vi "Auto.vi"() -> ()   [LabVIEW 2020]
uses:
  <vilib>/Utility/miscctls.llb/LVRowAndColumnTypeDef.ctl
  Global_Variable/Global.vi
  Global_Variable/A131258.vi
  Database/Global1.vi
  <vilib>/addons/database/Connection.llb/DB Tools Open Connec (String).vi
  <vilib>/addons/database/Connection.llb/Conn Execute.vi
  <vilib>/addons/database/Recordset.llb/Rec Fetch Recordset Data (R).vi
  <vilib>/addons/database/NI_Database_API.lvlib
panel:
  out "标尺_Event":refnum<user-event>
  out "判定完成":bool=TRUE
  out "采集初始化":bool=TRUE
  out "左code":string
  out "初始化":bool[](array[boolean])
  out "空载":cluster{dbl[], dbl[]}[](graph)
  in  "判定结果":bool[][](array[boolean])=[[TRUE]]
  in  "STEP":string
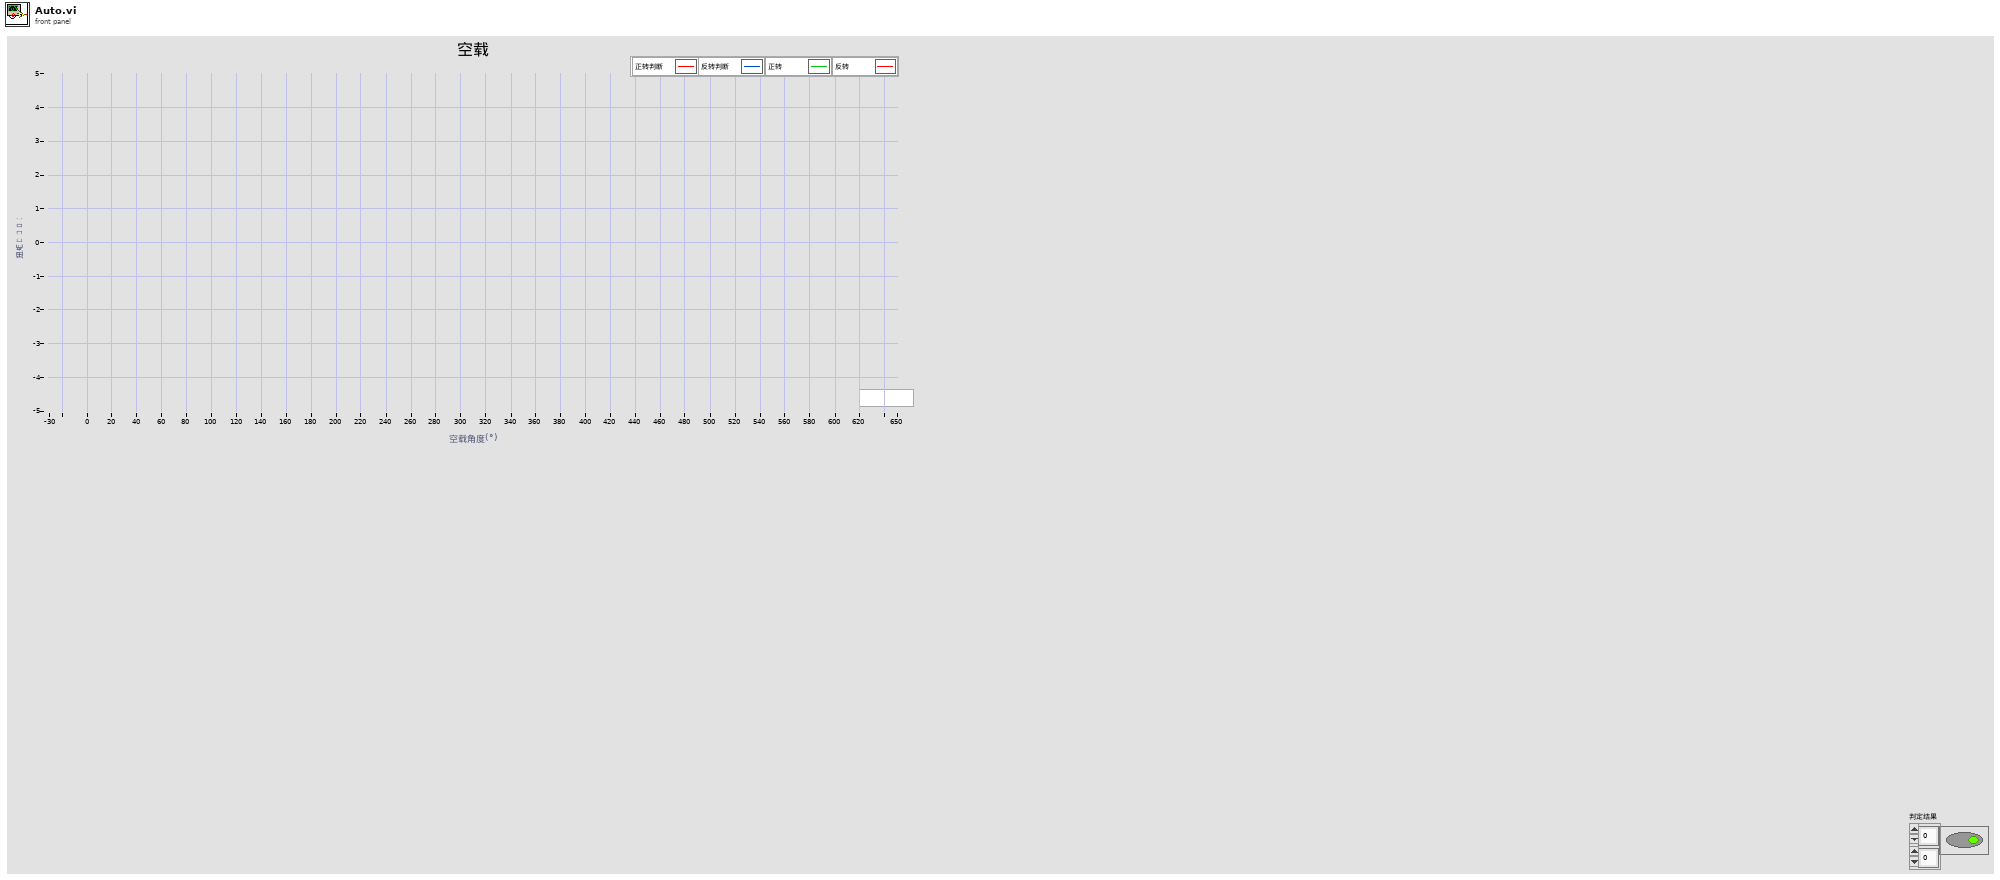
[diagram p1: front panel]
types:
  T1 = enum32{"Invalid", "Standard", "Closed", "Hidden", "Minimized", "Maximized"}
  T2 = typedef "LVRowAndColumnTypeDef.ctl" = cluster{"Row":i32, "Column":i32}
  T3 = typedef "lveventtype.ctl" = enum32{"Null", "Timeout", "Annotation Menu Selection", "Annotation Menu Selection?", "App Instance Close", "App Instance Close?", "Autoscale Range Change", "Bookmark Info Change", "Cell Edit", "Cell Edit?", "Cursor Grab", "Cursor Grab?", "Cursor Menu Selection", "Cursor Menu Selection?", "Cursor Move", "Cursor Release", "Data Change", "Direction Change", "Display State Change", "Drag Ended", "Drag Enter", "Drag Leave", "Drag Over", "Drag Source Update", "Drag Starting", "Drag Starting?", "Drop", "Exec State Change", "Key Down", "Key Down?", "Key Repeat", "Key Repeat?", "Key Up", "Listbox Double Click", "Menu Activation?", "Menu Selection (App)", "Menu Selection? (App)", "Menu Selection (User)", "Mouse Down", "Mouse Down?", "Mouse Enter", "Mouse Leave", "Mouse Move", "Mouse Up", "Mouse Wheel", "NI Security User Change (App)", "Pane Size", "Panel Close", "Panel Close?", "Panel Resize", "Plot Attribute Change", "Scale Range Change", "Shortcut Menu Activation?", "Shortcut Menu Selection (App)", "Shortcut Menu Selection? (App)", "Shortcut Menu Selection (User)", "Tree Double Click", "Tree Drag", "Tree Drag?", "Tree Drop", "Tree Drop?", "Tree Item Close", "Tree Item Close?", "Tree Item Open", "Tree Item Open?", "User Event", "Value Change"}
  T4 = typedef "LVPoint32TypeDef.ctl" = cluster{"Horizontal":i32, "Vertical":i32}
  T5 = cluster{"扭矩判定":cluster{"单位":string, "下限":dbl, "上限":dbl}, "正转扭矩最大值":cluster{"单位":string, "下限":dbl, "上限":dbl}, "正转扭矩最小值":cluster{"单位":string, "下限":dbl, "上限":dbl}, "正转扭矩波动值":cluster{"单位":string, "下限":dbl, "上限":dbl}, "正转平均扭矩值":cluster{"单位":string, "下限":dbl, "上限":dbl}, "反转扭矩最大值":cluster{"单位":string, "下限":dbl, "上限":dbl}, "反转扭矩最小值":cluster{"单位":string, "下限":dbl, "上限":dbl}, "反转扭矩波动值":cluster{"单位":string, "下限":dbl, "上限":dbl}, "反转扭矩平均值":cluster{"单位":string, "下限":dbl, "上限":dbl}, "正/逆转平均扭矩差":cluster{"单位":string, "下限":dbl, "上限":dbl}}
  T6 = cluster{"正向判定X值":cluster{"单位":string, "下限":dbl, "上限":dbl}, "正向判定Y值":cluster{"单位":string, "下限":dbl, "上限":dbl}, "逆向判定X值":cluster{"单位":string, "下限":dbl, "上限":dbl}, "逆向判定Y值":cluster{"单位":string, "下限":dbl, "上限":dbl}}
  T7 = cluster{"左平均扭矩":cluster{"正转":dbl, "反转":dbl}, "左矩波动":cluster{"正转":dbl, "反转":dbl}, "左空载":cluster{"正转":dbl, "反转":dbl}, "右平均扭矩":cluster{"正转":dbl, "反转":dbl}, "右扭矩波动":cluster{"正转":dbl, "反转":dbl}, "右空载":cluster{"正转":dbl, "反转":dbl}, "扭矩对称":cluster{"左":dbl, "右":dbl}, "左零点漂移":cluster{"正":dbl, "反":dbl}, "右零点漂移":cluster{"正":dbl, "反":dbl}}
  T8 = typedef "NI_Database_API.lvlib/Conn ObjectReference.ctl" = refnum<k1>
  T9 = typedef "NI_Database_API.lvlib/Rec ObjectReference.ctl" = refnum<k1>
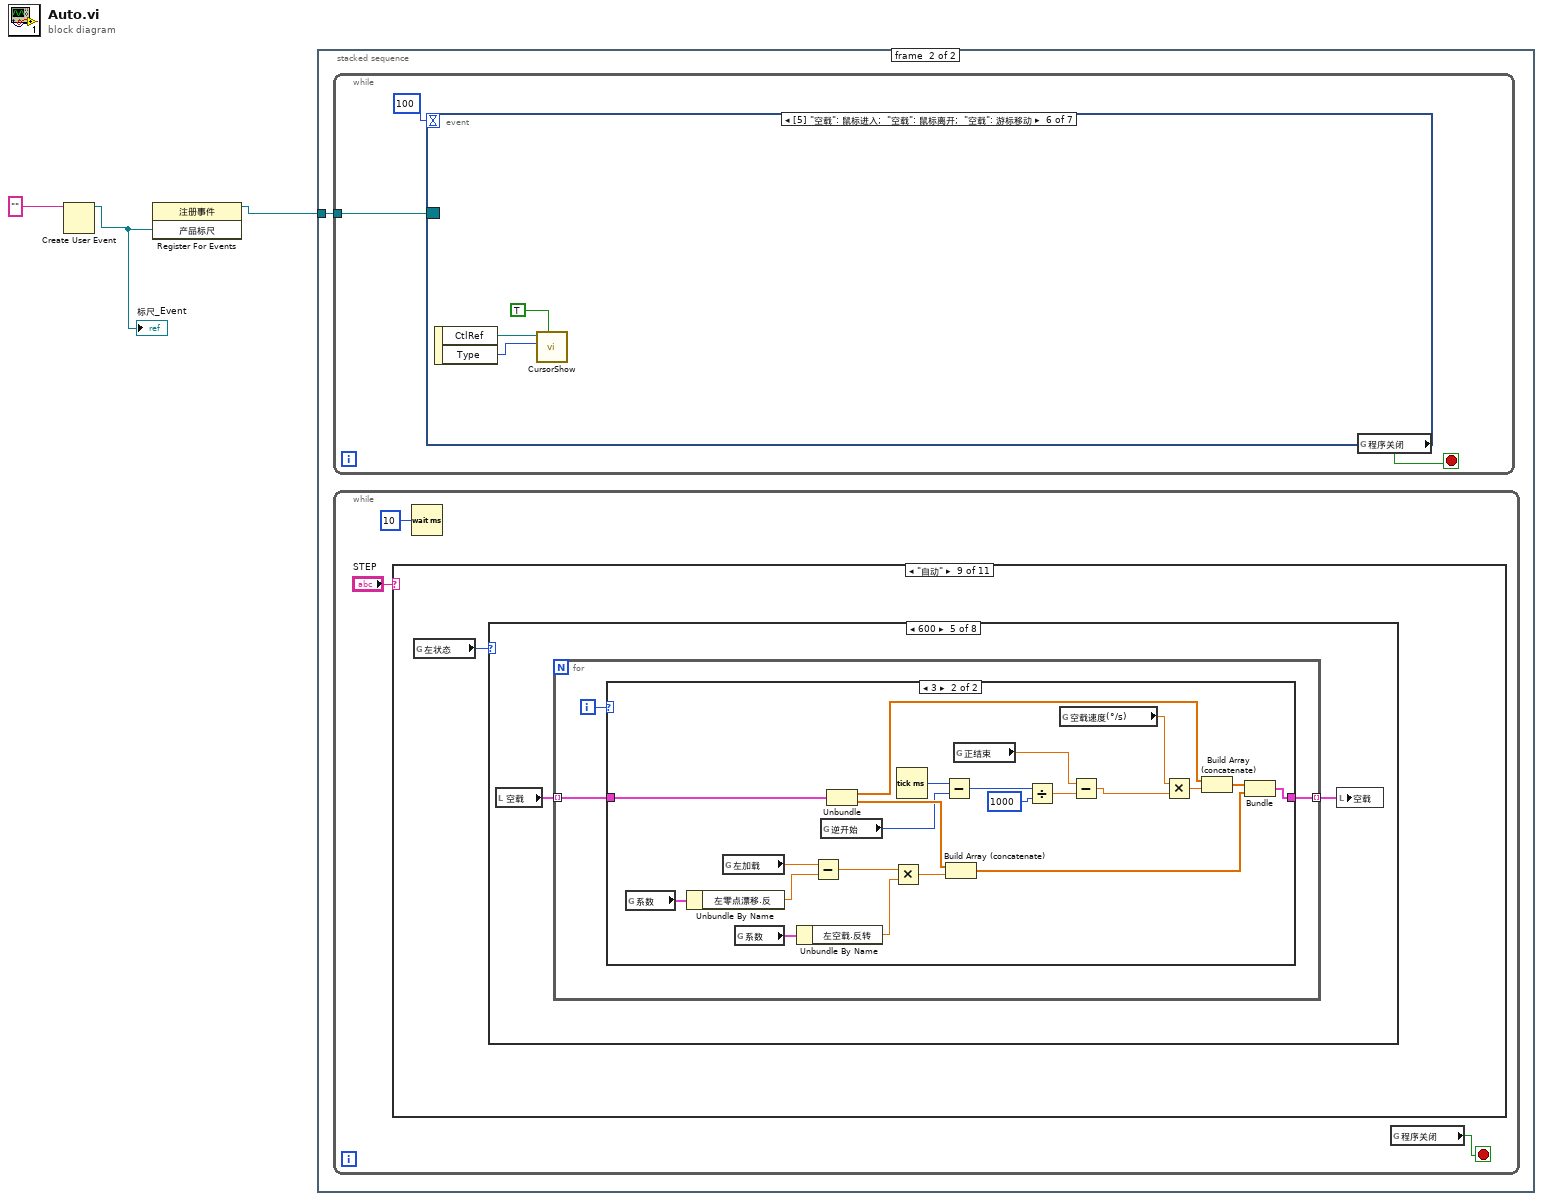
[diagram p0: block diagram]
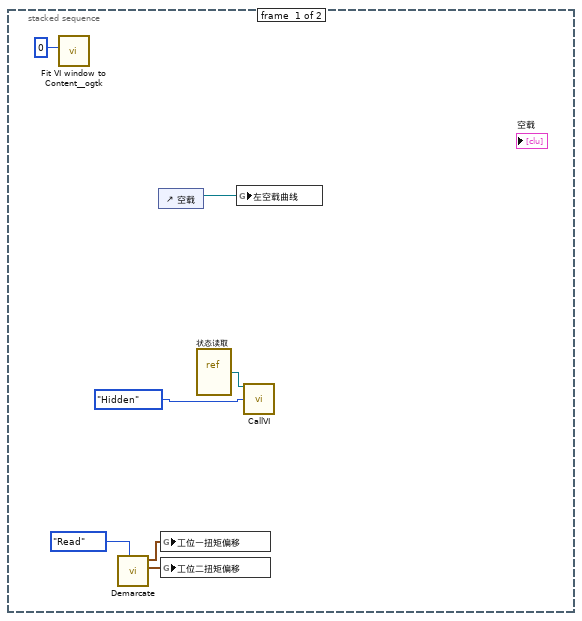
[diagram p2: hidden frame]
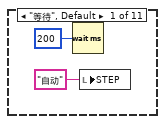
[diagram p3: hidden frame]
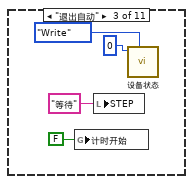
[diagram p5: hidden frame]
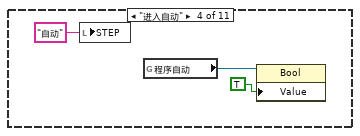
[diagram p6: hidden frame]
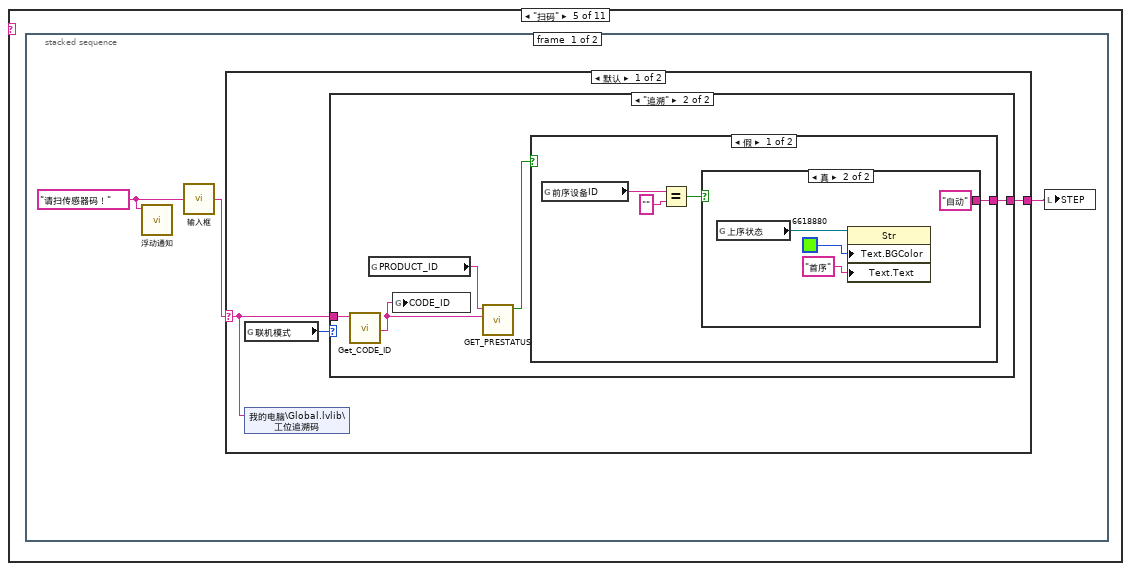
[diagram p7: hidden frame]
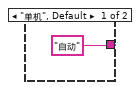
[diagram p8: hidden frame]
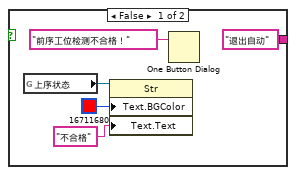
[diagram p9: hidden frame]
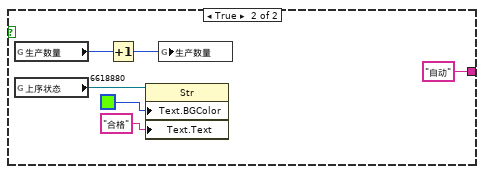
[diagram p10: hidden frame]
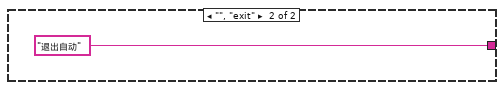
[diagram p11: hidden frame]
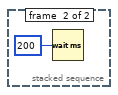
[diagram p12: hidden frame]
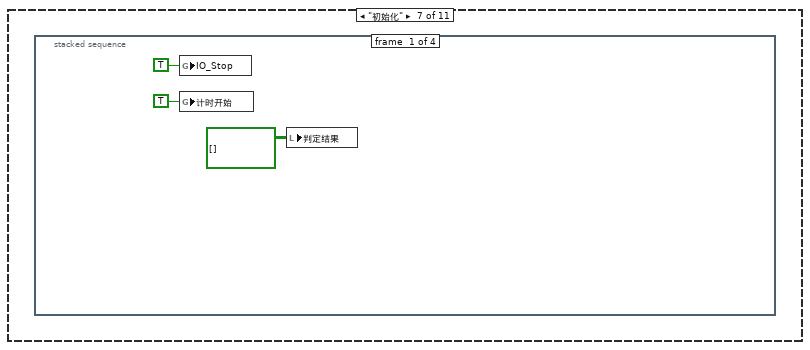
[diagram p14: hidden frame]
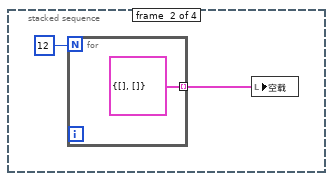
[diagram p15: hidden frame]
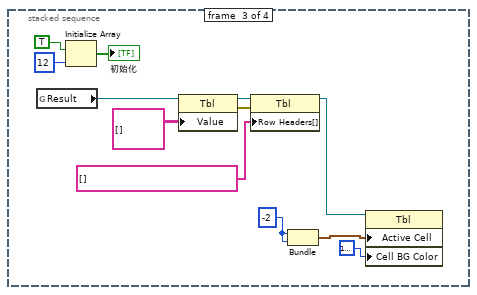
[diagram p16: hidden frame]
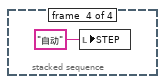
[diagram p17: hidden frame]
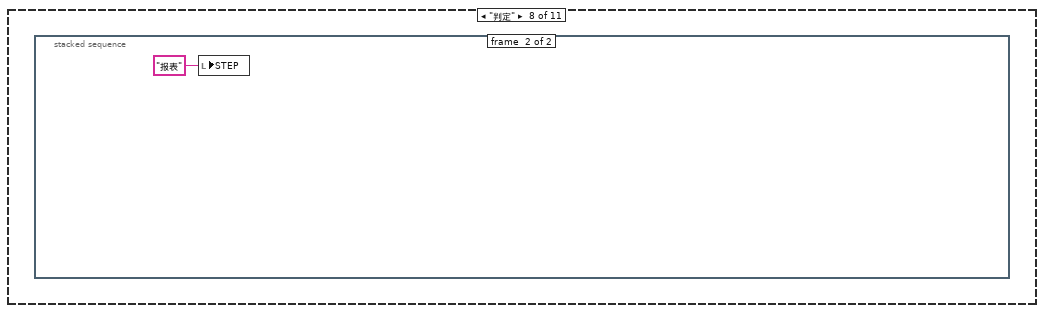
[diagram p18: hidden frame]
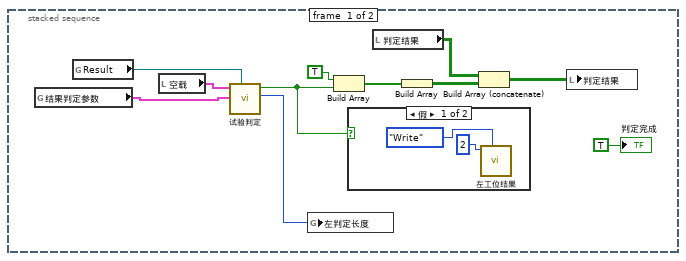
[diagram p19: hidden frame]
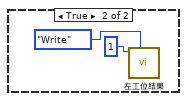
[diagram p20: hidden frame]
diagram:
  n1 = Create User Event(user event datatype="" ("产品标尺")) -> (user event=w2:refnum<user-event>)  [unwired: 1 in, 1 out]
  "标尺_Event" <- w2
  n2 = register-events(w2) -> (reference out=w1:refnum<event-registration>)  [unwired: 2 in, 1 out]
  n3 = stacked-sequence {
    tunnel: w1 -> [_ w11]
    frame #0 {
      n4 = call <userlib>:"Fit VI window to Content__ogtk.vi"("border spacing (2 px)"=0) -> ()  [unwired: 5 in, 2 out]
      n5 = call "Demarcate.vi"("Mode"=enum16{"Read", "Write"}."Read") -> ("工位二扭矩偏移O"=w5:cluster{"正向":dbl, "逆向":dbl}, "工位一扭矩偏移O"=w6:cluster{"正向":dbl, "逆向":dbl})  [unwired: 8 in, 1 out]
      n6 = control-ref of="空载"() -> (w4:refnum<vi>)
      n7 = global write "Global.vi" "工位一扭矩偏移"(w6) -> ()
      n8 = global write "Global.vi" "工位二扭矩偏移"(w5) -> ()
      n9 = vi-ref "状态读取.vi"() -> (w9:refnum<vi>)
      n10 = global write "A131258.vi" "左空载曲线"(w4) -> ()
      n11 = call "CallVI.vi"("VI引用"=w9, "状态"=T1."Hidden") -> ()  [unwired: 11 in, 3 out]
    }
    frame #1 {
      n12 = while {
        tunnel: w11 -> [w327]
        stop <- w328 stop-if-true
        n13 = event shown="[5] \"空载\": 鼠标进入;  \"空载\": 鼠标离开;  \"空载\": 游标移动" {
          selector: w327 -> [_ _ _ _ _ _ _]
          dyn-events: _ -> [_ _ _ _ _ _ _]
          timeout: 100 -> [_ _ _ _ _ _ _]
          event Timeout {
            n14 = event-data() -> ()  [unwired: 1 in, 3 out]
            n15 = global read "Global.vi" "跳转"() -> (w330:i16)
            n16 = case shown="1001" w330 {
              frame 0, Default {
              }
              frame 1000 {
                w334 = "" ("文本.文本")
                n17 = shared-variable "我的电脑\\Global.lvlib\\总成追溯码"(w334) -> ()  [unwired: 1 in, 1 out]
                n18 = shared-variable "我的电脑\\Global.lvlib\\工位追溯码"(w334) -> ()  [unwired: 1 in, 1 out]
                n19 = shared-variable "我的电脑\\Global.lvlib\\传感器码-左"(w334) -> ()  [unwired: 1 in, 1 out]
                n20 = shared-variable "我的电脑\\Global.lvlib\\传感器码-右"(w334) -> ()  [unwired: 1 in, 1 out]
                n21 = local write "STEP"("扫码" ("STEP")) -> ()
                n22 = call "跳转步骤.vi"("枚举"=enum16{"Read", "Write"}."Write", "Status_Write"=u16 1001 ("跳转步骤")) -> ()  [unwired: 9 in, 1 out]
              }
              frame 1001 {
                n23 = global read "Global.vi" "左在位"() -> (w335:i16)
                n24 = case shown="1" w335 {
                  frame 0, Default {
                  }
                  frame 1 {
                    w338 = enum16{"Read", "Write"}."Write" ("枚举")
                    n25 = local write "STEP"("自动" ("STEP")) -> ()
                    n26 = call "左工位状态.vi"("枚举"=w338, "Status_Write"=u16 1001 ("左工位状态")) -> ()  [unwired: 9 in, 1 out]
                    n27 = call "左工位在位.vi"("枚举"=w338, "Status_Write"=u16 0 ("左工位工件在位")) -> ()  [unwired: 9 in, 1 out]
                  }
                }
              }
            }
          }
          event Menu Selection (User) {
            n28 = event-data() -> ("ItemTag"=w340:string)  [unwired: 1 in, 2 out]
            n29 = case shown="\"假\", 默认" w340 {
              frame "假", Default {
              }
              frame "真" {
              }
            }
          }
          event "空载": Scale Range Change {
            n30 = event-data() -> ("CtlRef"=w343:refnum<vi>)  [unwired: 1 in]
            n31 = shared-variable "我的电脑\\Global.lvlib\\产品型号"() -> (w341:string)  [unwired: 1 in, 1 out]
            n32 = call "XY_conf.vi"("方式"=enum16{"写入", "读取"}."写入", "产品型号"=w341, "XY图引用"=w343) -> ()  [unwired: 3 in, 1 out]
          }
          event User Event {
            n33 = event-data() -> ("产品标尺"=w346:string)  [unwired: 1 in, 4 out]
            n34 = control-ref of="空载"() -> (w344:refnum<vi>)
            n35 = call "XY_conf.vi"("方式"=enum16{"写入", "读取"}."读取", "产品型号"=w346, "XY图引用"=w344) -> ()  [unwired: 3 in, 1 out]
          }
          event Panel Close {
            n36 = event-data() -> ()  [unwired: 1 in, 4 out]
            n37 = global write "Global.vi" "程序关闭"(TRUE ("程序关闭")) -> ()
          }
          event "空载": Mouse Enter; "空载": Mouse Leave; "空载": Cursor Move {
            n38 = event-data() -> ("CtlRef"=w350:refnum<vi>, "Type"=w348:T3)  [unwired: 1 in]
            n39 = call "CursorShow.vi"("nameShow"=TRUE, "Type"=w348, "Graph"=w350) -> ()  [unwired: 7 in, 2 out]
          }
          event "空载": Mouse Down {
            n40 = event-data() -> ("CtlRef"=w355:refnum<vi>, "Coords"=w354:T4, "Type"=w352:T3)  [unwired: 1 in]
            n41 = invoke class="XYGraph (严格)" method="Map Coords To XY"(reference=w355, "Coords"=w354) -> (reference out=w353:refnum<vi>, "XY"=w351:cluster{"X":dbl, "Y":dbl})  [unwired: 5 in, 5 out]
            n42 = call "CursorShow.vi"("游标.游标位置"=w351, "Type"=w352, "Graph"=w353) -> ()  [unwired: 7 in, 2 out]
          }
        }
        n43 = global read "Global.vi" "程序关闭"() -> (w328:bool)
      }
      n44 = while {
        stop <- w14 stop-if-true
        n45 = case shown="\"自动\"" "STEP" {
          frame "等待", Default {
            n46 = Wait (ms)(milliseconds to wait=u32 200 ("等待时间（毫秒）")) -> ()  [unwired: 1 out]
            n47 = local write "STEP"("自动" ("STEP")) -> ()
          }
          frame "手动" {
          }
          frame "退出自动" {
            n48 = global write "Global.vi" "计时开始"(FALSE ("计时开始")) -> ()
            n49 = local write "STEP"("等待" ("STEP")) -> ()
            n50 = call "设备状态.vi"("枚举"=enum16{"Read", "Write"}."Write", "Status_Write"=i16 0) -> ()  [unwired: 9 in, 1 out]
          }
          frame "进入自动" {
            n51 = local write "STEP"("自动" ("STEP")) -> ()
            n52 = global read "Global.vi" "程序自动"() -> (w22:refnum<vi>)
            n53 = property class="Bool"(reference=w22, "Value"=TRUE) -> ()  [unwired: 1 in, 2 out]
          }
          frame "扫码" {
            n54 = stacked-sequence {
              frame #0 {
                w25 = "请扫传感器码！" ("提示信息")
                n55 = call "浮动通知.vi"("通知内容"=w25) -> ()  [unwired: 11 in]
                n56 = call "输入框.vi"("提示信息"=w25) -> ("条形码输出"=w26:string)
                n57 = case shown="默认" w26 {
                  selector: w26 -> [w27 _]
                  tunnel: [w29 "退出自动" ("State(s) in Front (\"\")")] -> w24
                  frame Default {
                    n58 = global read "Global1.vi" "联机模式"() -> (w28:enum16{"单机", "追溯"})
                    n59 = shared-variable "我的电脑\\Global.lvlib\\工位追溯码"(w27) -> ()  [unwired: 1 in, 1 out]
                    n60 = case shown="\"追溯\"" w28 {
                      tunnel: ["自动" ("State(s) in Front (\"\")") w35] -> w29
                      tunnel: w27 -> [_ w34]
                      frame "单机", Default {
                      }
                      frame "追溯" {
                        n61 = call "Get_CODE_ID.vi"("CODE_MAIN"=w34) -> ("CODE_ID"=w31:string)  [unwired: 10 in]
                        n62 = global read "追溯Global.vi" "PRODUCT_ID"() -> (w33:string)
                        n63 = global write "追溯Global.vi" "CODE_ID"(w31) -> ()
                        n64 = call "GET_PRESTATUS.vi"("CODE_ID"=w31, "PRODUCT_ID"=w33) -> ("OK?"=w32:bool)  [unwired: 8 in, 1 out]
                        n65 = case shown="假" w32 {
                          tunnel: [w39 "自动" ("State(s) in Front (\"\")")] -> w35
                          frame False {
                            n66 = global read "追溯Global.vi" "前序设备ID"() -> (w38:string)
                            n67 = Equal?(x=w38, y="") -> (x = y?=w37:bool)
                            n68 = case shown="真" w37 {
                              tunnel: ["退出自动" ("State(s) in Front (\"\")") "自动" ("State(s) in Front (\"\")")] -> w39
                              frame False {
                                n69 = global read "Global.vi" "上序状态"() -> (w42:refnum<vi>)
                                n70 = property class="Str"(reference=w42, "Text.BGColor"=u32 16711680 ("文本.文本颜色:背景色"), "Text.Text"="不合格" ("文本.文本")) -> ()  [unwired: 1 in, 2 out]
                                n71 = One Button Dialog(message="前序工位检测不合格！" ("消息")) -> ()  [unwired: 1 in, 1 out]
                              }
                              frame True {
                                n72 = global read "Global.vi" "上序状态"() -> (w47:refnum<vi>)
                                n73 = property class="Str"(reference=w47, "Text.BGColor"=u32 6618880 ("文本.文本颜色:背景色"), "Text.Text"="首序" ("文本.文本")) -> ()  [unwired: 1 in, 2 out]
                              }
                            }
                          }
                          frame True {
                            n74 = global read "Global.vi" "生产数量"() -> (w52:i32)
                            n75 = global read "Global.vi" "上序状态"() -> (w51:refnum<vi>)
                            n76 = Increment(x=w52) -> (x+1=w53:i32)
                            n77 = property class="Str"(reference=w51, "Text.BGColor"=u32 6618880 ("文本.文本颜色:背景色"), "Text.Text"="合格" ("文本.文本")) -> ()  [unwired: 1 in, 2 out]
                            n78 = global write "Global.vi" "生产数量"(w53) -> ()
                          }
                        }
                      }
                    }
                  }
                  frame "", "exit" {
                  }
                }
                n79 = local write "STEP"(w24) -> ()
              }
              frame #1 {
                n80 = Wait (ms)(milliseconds to wait=u32 200 ("等待时间（毫秒）")) -> ()  [unwired: 1 out]
              }
            }
          }
          frame "工位判断" {
          }
          frame "初始化" {
            n81 = stacked-sequence {
              frame #0 {
                n82 = global write "Global.vi" "IO_Stop"(TRUE ("IO_Stop")) -> ()
                n83 = global write "Global.vi" "计时开始"(TRUE ("计时开始")) -> ()
                n84 = local write "判定结果"(bool[][] [] ("判定结果")) -> ()
              }
              frame #1 {
                n85 = for {
                  N: 12 -> [_]
                  tunnel: [cluster{dbl[], dbl[]} {[], []}] -> w60 mode=indexing
                }
                n86 = local write "空载"(w60) -> ()
              }
              frame #2 {
                w63 = -2 ("维数大小")
                n87 = global read "Global.vi" "Result"() -> (w72:refnum<vi>)
                n88 = Initialize Array(TRUE, 12 ("维数大小")) -> (→"初始化":bool[])
                n89 = property class="Tbl"(reference=w72, "Value"=string[][] []) -> (reference out=w73:refnum<vi>, error out=w74:errorcluster)  [unwired: 1 in]
                n90 = property class="Tbl"(reference=w73, error in=w74, "Row Headers[]"=string[] [] ("列首字符串[]")) -> (reference out=w66:refnum<vi>)  [unwired: 1 out]
                n91 = Bundle("维数大小"=w63, "维数大小"=w63) -> (w64:cluster{"维数大小":i32, "维数大小":i32})  [unwired: 1 in]
                n92 = property class="Tbl"(reference=w66, "Active Cell"=w64, "Cell BG Color"=u32 16777216 ("活动单元格:单元格背景色")) -> ()  [unwired: 1 in, 2 out]
              }
              frame #3 {
                n93 = local write "STEP"("自动" ("STEP")) -> ()
              }
            }
          }
          frame "判定" {
            n94 = stacked-sequence {
              frame #0 {
                n95 = global read "A131258.vi" "结果判定参数"() -> (w78:T5)
                n96 = global read "Global.vi" "Result"() -> (w80:refnum<vi>)
                n97 = local read "空载"() -> (w79:cluster{dbl[], dbl[]}[])
                n98 = call "试验判定.vi"("Result"=w80, "判定参数"=w78, "XY曲线"=w79) -> ("判定项长度"=w77:i32, "OK？"=w81:bool)  [unwired: 7 in]
                n99 = global write "判定参数.vi" "左判定长度"(w77) -> ()
                n100 = Build Array(TRUE ("元素"), w81) -> (w84:bool[])
                n101 = case shown="假" w81 {
                  frame False {
                    n102 = call "左工位结果.vi"("枚举"=enum16{"Read", "Write"}."Write", "Status_Write"=u16 2 ("左工位生产结果")) -> ()  [unwired: 9 in, 1 out]
                  }
                  frame True {
                    n103 = call "左工位结果.vi"("枚举"=enum16{"Read", "Write"}."Write", "Status_Write"=u16 1 ("左工位生产结果")) -> ()  [unwired: 9 in, 1 out]
                  }
                }
                n104 = local read "判定结果"() -> (w85:bool[][])
                n105 = Build Array(w84) -> (w83:bool[][])
                n106 = Build Array (concatenate)(w85, w83) -> (w86:bool[][])
                n107 = local write "判定结果"(w86) -> ()
                "判定完成" <- TRUE
              }
              frame #1 {
                n108 = local write "STEP"("报表" ("STEP")) -> ()
              }
            }
          }
          frame "自动" {
            n109 = global read "Global.vi" "左状态"() -> (w92:i16)
            n110 = case shown="600" w92 {
              frame 0, Default {
              }
              frame 3 {
                n111 = stacked-sequence {
                  frame #0 {
                    n112 = local write "判定结果"(bool[][] [] ("判定结果")) -> ()
                    n113 = call "左工位结果.vi"("枚举"=enum16{"Read", "Write"}."Write", "Status_Write"=i16 0) -> ()  [unwired: 9 in, 1 out]
                  }
                  frame #1 {
                    n114 = global read "Global.vi" "空载速度(°/s) 2"() -> (w96:sgl)
                    n115 = Multiply(x=w96, y=sgl 6.0) -> (x*y=w97:sgl)
                    n116 = global write "Global.vi" "空载速度(°/s)"(w97) -> ()
                  }
                }
              }
              frame 200 {
                n117 = stacked-sequence {
                  frame #0 {
                    n118 = local write "判定完成"(FALSE ("判定完成")) -> ()
                    n119 = call "左工位结果.vi"("枚举"=enum16{"Read", "Write"}."Write", "Status_Write"=u16 0 ("左工位生产结果")) -> ()  [unwired: 9 in, 1 out]
                    "采集初始化" <- TRUE
                  }
                  frame #1 {
                    n120 = for {
                      N: 4 -> [_]
                      tunnel: [cluster{dbl[], dbl[]} {[], []}] -> w104 mode=indexing
                    }
                    n121 = local write "空载"(w104) -> ()
                  }
                  frame #2 {
                    n122 = global read "Global.vi" "Result"() -> (w110:refnum<vi>)
                    n123 = property class="Tbl"(reference=w110, "Row Headers[]"=string[] [] ("行首字符串[]"), "Value"=string[][] [] ("值"), "Active Cell"=T2 {"Row"=-2, "Column"=-2} ("活动单元格:活动单元格"), "Cell BG Color"=u32 16777216 ("活动单元格:单元格背景色")) -> ()  [unwired: 1 in, 2 out]
                  }
                  frame #3 {
                    n124 = local read "空载"() -> (w111:cluster{dbl[], dbl[]}[])
                    n125 = for {
                      tunnel: [w114] -> w112 mode=indexing
                      tunnel: w111 -> [w113] mode=indexing
                      i -> [w115]
                      n126 = case shown="1" w115 {
                        tunnel: [w116 w117 w125] -> w114
                        tunnel: w113 -> [w116 _ _]
                        frame Default {
                        }
                        frame 0 {
                          n127 = global read "A131258.vi" "判定框参数"() -> (w122:T6)
                          n128 = Unbundle By Name(w122) -> ("正向判定X值.下限"=w121:dbl, "正向判定X值.上限"=w120:dbl, "正向判定Y值.下限"=w119:dbl, "正向判定Y值.上限"=w118:dbl)
                          n129 = Build Array(w120, w120, w121, w121, w120) -> (w124:dbl[])
                          n130 = Build Array(w118, w119, w119, w118, w118) -> (w123:dbl[])
                          n131 = Bundle(w124, w123) -> (w117:cluster{dbl[], dbl[]})  [unwired: 1 in]
                        }
                        frame 1 {
                          n132 = global read "A131258.vi" "判定框参数"() -> (w130:T6)
                          n133 = Unbundle By Name(w130) -> ("逆向判定X值.下限"=w129:dbl, "逆向判定X值.上限"=w128:dbl, "逆向判定Y值.下限"=w127:dbl, "逆向判定Y值.上限"=w126:dbl)
                          n134 = Build Array(w128, w128, w129, w129, w128) -> (w132:dbl[])
                          n135 = Build Array(w126, w127, w127, w126, w126) -> (w131:dbl[])
                          n136 = Bundle(w132, w131) -> (w125:cluster{dbl[], dbl[]})  [unwired: 1 in]
                        }
                      }
                    }
                    n137 = local write "空载"(w112) -> ()
                  }
                  frame #4 {
                    n138 = call "左工位状态.vi"("枚举"=enum16{"Read", "Write"}."Write", "Status_Write"=u16 500 ("左工位状态")) -> ()  [unwired: 9 in, 1 out]
                  }
                }
              }
              frame 500 {
                n139 = local read "空载"() -> (w136:cluster{dbl[], dbl[]}[])
                n140 = for {
                  tunnel: w136 -> [w138] mode=indexing
                  tunnel: [w137] -> w135 mode=indexing
                  i -> [w139]
                  n141 = case shown="2" w139 {
                    tunnel: w138 -> [w140 w155]
                    tunnel: [w140 w148] -> w137
                    frame Default {
                    }
                    frame 2 {
                      n142 = local read "采集初始化"() -> (w141:bool)
                      n143 = Unbundle(w155) -> (w150:dbl[], w154:dbl[])
                      n144 = global read "A131258.vi" "系数"() -> (w144:T7)
                      n145 = global read "A131258.vi" "系数"() -> (w157:T7)
                      n146 = Unbundle By Name(w144) -> ("左零点漂移.正"=w143:dbl)
                      n147 = Unbundle By Name(w157) -> ("左空载.正转"=w156:dbl)
                      n148 = case shown="真" w141 {
                        tunnel: [w158 0.0] -> w142
                        frame False {
                          n149 = global read "全局 1.vi" "正开始"() -> (w162:u32)
                          n150 = Tick Count (ms)() -> (millisecond timer value=w159:u32)
                          n151 = Subtract(x=w159, y=w162) -> (x-y=w161:u32)
                          n152 = global write "全局 1.vi" "逆开始"(w159) -> ()
                          n153 = Divide(x=w161, y=u32 1000) -> (x/y=w158:dbl)
                        }
                        frame True {
                          n154 = Tick Count (ms)() -> (millisecond timer value=w163:u32)
                          n155 = local write "采集初始化"(FALSE ("采集初始化")) -> ()
                          n156 = global write "全局 1.vi" "正开始"(w163) -> ()
                        }
                      }
                      n157 = global read "全局1.vi" "左加载"() -> (w145:dbl)
                      n158 = Subtract(x=w145, y=w143) -> (x-y=w146:dbl)
                      n159 = Multiply(x=w146, y=w156) -> (x*y=w153:dbl)
                      n160 = Build Array (concatenate)(w154, w153) -> (w147:dbl[])
                      n161 = global read "Global.vi" "空载速度(°/s)"() -> (w152:sgl)
                      n162 = global write "全局 1.vi" "正结束"(w142) -> ()
                      n163 = Multiply(x=w152, y=w142) -> (x*y=w151:dbl)
                      n164 = Build Array (concatenate)(w150, w151) -> (w149:dbl[])
                      n165 = Bundle(w149, w147) -> (w148:cluster{dbl[], dbl[]})  [unwired: 1 in]
                    }
                  }
                }
                n166 = local write "空载"(w135) -> ()
              }
              frame 600 {
                n167 = local read "空载"() -> (w167:cluster{dbl[], dbl[]}[])
                n168 = for {
                  tunnel: w167 -> [w169] mode=indexing
                  tunnel: [w168] -> w166 mode=indexing
                  i -> [w170]
                  n169 = case shown="3" w170 {
                    tunnel: w169 -> [w171 w191]
                    tunnel: [w171 w182] -> w168
                    frame 0, Default {
                    }
                    frame 3 {
                      n170 = global read "A131258.vi" "系数"() -> (w179:T7)
                      n171 = Unbundle By Name(w179) -> ("左零点漂移.反"=w178:dbl)
                      n172 = global read "全局1.vi" "左加载"() -> (w181:dbl)
                      n173 = global read "A131258.vi" "系数"() -> (w193:T7)
                      n174 = Unbundle By Name(w193) -> ("左空载.反转"=w192:dbl)
                      n175 = Subtract(x=w181, y=w178) -> (x-y=w180:dbl)
                      n176 = global read "全局 1.vi" "逆开始"() -> (w177:u32)
                      n177 = Unbundle(w191) -> (w185:dbl[], w190:dbl[])
                      n178 = Multiply(x=w180, y=w192) -> (x*y=w189:dbl)
                      n179 = Tick Count (ms)() -> (millisecond timer value=w176:u32)
                      n180 = Subtract(x=w176, y=w177) -> (x-y=w175:u32)
                      n181 = Build Array (concatenate)(w190, w189) -> (w183:dbl[])
                      n182 = global read "全局 1.vi" "正结束"() -> (w173:dbl)
                      n183 = Divide(x=w175, y=u32 1000) -> (x/y=w172:dbl)
                      n184 = global read "Global.vi" "空载速度(°/s)"() -> (w187:sgl)
                      n185 = Subtract(x=w173, y=w172) -> (x-y=w188:dbl)
                      n186 = Multiply(x=w187, y=w188) -> (x*y=w186:dbl)
                      n187 = Build Array (concatenate)(w185, w186) -> (w184:dbl[])
                      n188 = Bundle(w184, w183) -> (w182:cluster{dbl[], dbl[]})  [unwired: 1 in]
                    }
                  }
                }
                n189 = local write "空载"(w166) -> ()
              }
              frame 650 {
                n190 = local read "判定完成"() -> (w194:bool)
                n191 = case shown="假" w194 {
                  frame False {
                    n192 = local write "STEP"("判定" ("STEP")) -> ()
                  }
                  frame True {
                  }
                }
                n193 = disable-structure shown="禁用" {
                  frame Disabled {
                    n194 = call "左工位状态.vi"("枚举"=enum16{"Read", "Write"}."Write", "Status_Write"=u16 1 ("左工位状态")) -> ()  [unwired: 9 in, 1 out]
                  }
                  frame Enabled {
                  }
                }
              }
              frame 1001 {
                n195 = stacked-sequence {
                  frame #0 {
                    n196 = shared-variable "我的电脑\\Global.lvlib\\工位追溯码"() -> (w198:string)  [unwired: 1 in, 1 out]
                    n197 = Wait (ms)(milliseconds to wait=u32 50 ("等待时间（毫秒）")) -> ()  [unwired: 1 out]
                    n198 = shared-variable "我的电脑\\Global.lvlib\\传感器码-左"(w198) -> ()  [unwired: 1 in, 1 out]
                  }
                  frame #1 {
                    n199 = global read "Global1.vi" "联机模式"() -> (w200:enum16{"单机", "追溯"})
                    n200 = case shown="\"追溯\"" w200 {
                      selector: w200 -> [_ w210]
                      frame "单机", Default {
                      }
                      frame "追溯" {
                        n201 = shared-variable "我的电脑\\Global.lvlib\\传感器码-左"() -> (w201:string)  [unwired: 1 in, 1 out]
                        n202 = global read "追溯Global.vi" "PRODUCT_ID"() -> (w207:string)
                        n203 = Bundle("String"=w201, "PRODUCT_ID"=w207) -> (w206:cluster{"String":string, "PRODUCT_ID":string})  [unwired: 1 in]
                        n204 = call "GetSQLstring.vi"("联机模式"=w210) -> ("错误输出"=w208:errorcluster, "连接字符串"=w209:string)  [unwired: 9 in]
                        n205 = Build Array(w206) -> (w202:cluster{"String":string, "PRODUCT_ID":string}[])
                        n206 = call-poly <vilib>:"DB Tools Open Connection.vi"("error in (no error)"=w208, "connection information"=w209) -> ("error out"=w204:errorcluster, "connection reference"=w205:T8)  [unwired: 6 in]
                        n207 = for {
                          tunnel: w205 -> [w218]
                          shift-right: [w215] -> w203
                          shift-left: w204 -> [w217]
                          tunnel: w202 -> [w211] mode=indexing
                          n208 = call <vilib>:"DB Tools Insert Data.vi"("data"=w211, "error in (no error)"=w217, "columns"=string[] ["CODE_SENSOR", "PRODUCT_ID"], "table"="Code", "connection reference"=w218) -> ("error out"=w216:errorcluster, "connection reference out"=w214:T8)  [unwired: 5 in]
                          n209 = case shown="错误 .." w216 {
                            selector: w216 -> [w220 w222]
                            tunnel: [w220 w223] -> w215
                            tunnel: [w219 w221] -> _
                            tunnel: w214 -> [w219 w221]
                            frame No Error {
                            }
                            frame Error {
                              n210 = call <vilib>:"Clear Errors.vi"("error in (no error)"=w222) -> ("error out"=w223:errorcluster)  [unwired: 5 in, 1 out]
                            }
                          }
                        }
                        n211 = call <vilib>:"Simple Error Handler.vi"("error in (no error)"=w203) -> ()  [unwired: 4 in, 5 out]
                      }
                    }
                  }
                  frame #2 {
                    n212 = global read "Global1.vi" "联机模式"() -> (w224:enum16{"单机", "追溯"})
                    n213 = case shown="\"追溯\"" w224 {
                      selector: w224 -> [_ w245]
                      frame "单机", Default {
                      }
                      frame "追溯" {
                        w237 = "'"
                        n214 = shared-variable "我的电脑\\Global.lvlib\\传感器码-左"() -> (w225:string)  [unwired: 1 in, 1 out]
                        n215 = global read "追溯Global.vi" "PRODUCT_ID"() -> (w238:string)
                        n216 = call "GetSQLstring.vi"("联机模式"=w245) -> ("错误输出"=w243:errorcluster, "连接字符串"=w244:string)  [unwired: 9 in]
                        n217 = Concatenate Strings("SELECT CODE_ID FROM CODE  WHERE CODE_SENSOR = '" ("table"), w225, w237, " AND PRODUCT_ID='" ("字符串"), w238, w237) -> (w236:string)
                        n218 = call-poly <vilib>:"DB Tools Open Connection.vi"("error in (no error)"=w243, "connection information"=w244) -> ("error out"=w242:errorcluster, "connection reference"=w241:T8)  [unwired: 6 in]
                        n219 = call-poly <vilib>:"DB Tools Execute Query.vi"("error in (no error)"=w242, "SQL query"=w236, "connection reference"=w241) -> ("error out"=w235:errorcluster, "recordset reference"=w234:T9)  [unwired: 5 in]
                        n220 = call-poly <vilib>:"DB Tools Fetch Recordset Data.vi"("error in (no error)"=w235, "recordset reference"=w234) -> ("error out"=w233:errorcluster, "recordset data"=w232:variant[][])  [unwired: 3 in, 1 out]
                        n221 = Variant To Data(error in=w233, type=string[][] [], Variant=w232) -> (data=w230:string[][])  [unwired: 1 out]
                        n222 = Index Array(array=w230, index (row)=0 ("索引 (行)")) -> (element=w229:string[])  [unwired: 1 in]
                        n223 = Index Array(array=w229, index=0 ("索引")) -> (element=→"左code":string)
                      }
                    }
                  }
                  frame #3 {
                    n224 = Wait (ms)(milliseconds to wait=u32 50 ("等待时间（毫秒）")) -> ()  [unwired: 1 out]
                    n225 = call "左工位状态.vi"("枚举"=enum16{"Read", "Write"}."Write", "Status_Write"=u16 1003 ("左工位状态")) -> ()  [unwired: 9 in, 1 out]
                  }
                }
              }
              frame 1002 {
                n226 = stacked-sequence {
                  frame #0 {
                    n227 = shared-variable "我的电脑\\Global.lvlib\\总成追溯码"() -> (w249:string)  [unwired: 1 in, 1 out]
                    n228 = shared-variable "我的电脑\\Global.lvlib\\传感器码-左"(w249) -> ()  [unwired: 1 in, 1 out]
                    n229 = Wait (ms)(milliseconds to wait=u32 100 ("等待时间（毫秒）")) -> ()  [unwired: 1 out]
                  }
                  frame #1 {
                    n230 = global read "Global1.vi" "联机模式"() -> (w251:enum16{"单机", "追溯"})
                    n231 = case shown="\"追溯\"" w251 {
                      selector: w251 -> [_ w261]
                      frame "单机", Default {
                      }
                      frame "追溯" {
                        n232 = shared-variable "我的电脑\\Global.lvlib\\传感器码-左"() -> (w252:string)  [unwired: 1 in, 1 out]
                        n233 = global read "追溯Global.vi" "PRODUCT_ID"() -> (w260:string)
                        n234 = Bundle("String"=w252, "PRODUCT_ID"=w260) -> (w258:cluster{"String":string, "PRODUCT_ID":string})  [unwired: 1 in]
                        n235 = call "GetSQLstring.vi"("联机模式"=w261) -> ("错误输出"=w257:errorcluster, "连接字符串"=w259:string)  [unwired: 9 in]
                        n236 = Build Array(w258) -> (w253:cluster{"String":string, "PRODUCT_ID":string}[])
                        n237 = call-poly <vilib>:"DB Tools Open Connection.vi"("error in (no error)"=w257, "connection information"=w259) -> ("error out"=w254:errorcluster, "connection reference"=w256:T8)  [unwired: 6 in]
                        n238 = for {
                          tunnel: w253 -> [w268] mode=indexing
                          tunnel: w256 -> [w267]
                          shift-right: [w263] -> w255
                          shift-left: w254 -> [w262]
                          n239 = call <vilib>:"DB Tools Insert Data.vi"("data"=w268, "error in (no error)"=w262, "columns"=string[] ["CODE_SENSOR", "PRODUCT_ID"], "table"="Code", "connection reference"=w267) -> ("error out"=w264:errorcluster)  [unwired: 5 in, 1 out]
                          n240 = case shown="无错误" w264 {
                            selector: w264 -> [w269 w270]
                            tunnel: [w269 w271] -> w263
                            frame No Error {
                            }
                            frame Error {
                              n241 = call <vilib>:"Clear Errors.vi"("error in (no error)"=w270) -> ("error out"=w271:errorcluster)  [unwired: 5 in, 1 out]
                            }
                          }
                        }
                        n242 = call <vilib>:"Simple Error Handler.vi"("error in (no error)"=w255) -> ()  [unwired: 4 in, 5 out]
                      }
                    }
                  }
                  frame #2 {
                    n243 = global read "Global1.vi" "联机模式"() -> (w272:enum16{"单机", "追溯"})
                    n244 = case shown="\"追溯\"" w272 {
                      selector: w272 -> [_ w293]
                      frame "单机", Default {
                      }
                      frame "追溯" {
                        w285 = "'"
                        n245 = shared-variable "我的电脑\\Global.lvlib\\传感器码-左"() -> (w273:string)  [unwired: 1 in, 1 out]
                        n246 = global read "追溯Global.vi" "PRODUCT_ID"() -> (w286:string)
                        n247 = call "GetSQLstring.vi"("联机模式"=w293) -> ("错误输出"=w291:errorcluster, "连接字符串"=w292:string)  [unwired: 9 in]
                        n248 = Concatenate Strings("SELECT CODE_ID FROM CODE  WHERE CODE_SENSOR = '" ("table"), w273, w285, " AND PRODUCT_ID='" ("字符串"), w286, w285) -> (w284:string)
                        n249 = call-poly <vilib>:"DB Tools Open Connection.vi"("error in (no error)"=w291, "connection information"=w292) -> ("error out"=w290:errorcluster, "connection reference"=w289:T8)  [unwired: 6 in]
                        n250 = call-poly <vilib>:"DB Tools Execute Query.vi"("error in (no error)"=w290, "SQL query"=w284, "connection reference"=w289) -> ("error out"=w283:errorcluster, "recordset reference"=w282:T9)  [unwired: 5 in]
                        n251 = call-poly <vilib>:"DB Tools Fetch Recordset Data.vi"("error in (no error)"=w283, "recordset reference"=w282) -> ("error out"=w281:errorcluster, "recordset data"=w280:variant[][])  [unwired: 3 in, 1 out]
                        n252 = Variant To Data(error in=w281, type=string[][] [], Variant=w280) -> (data=w278:string[][])  [unwired: 1 out]
                        n253 = Index Array(array=w278, index (row)=0 ("索引 (行)")) -> (element=w277:string[])  [unwired: 1 in]
                        n254 = Index Array(array=w277, index=0 ("索引")) -> (element=w276:string)
                        n255 = local write "左code"(w276) -> ()
                      }
                    }
                  }
                  frame #3 {
                    n256 = local write "STEP"("自动" ("STEP")) -> ()
                    n257 = call "左工位状态.vi"("枚举"=enum16{"Read", "Write"}."Write", "Status_Write"=u16 1003 ("左工位状态")) -> ()  [unwired: 9 in, 1 out]
                  }
                }
              }
            }
          }
          frame "不合格" {
            n258 = Wait (ms)(milliseconds to wait=u32 100 ("等待时间（毫秒）")) -> ()  [unwired: 1 out]
            n259 = local write "STEP"("等待" ("STEP")) -> ()
          }
          frame "报表" {
            n260 = global read "Global.vi" "左启用"() -> (w299:i16)
            n261 = case shown="1" w299 {
              frame 0, Default {
              }
              frame 1 {
                n262 = stacked-sequence {
                  frame #0 {
                    n263 = stacked-sequence {
                      seq-local: [w302 _ _] -> [_ w305 _]
                      frame #0 {
                        n264 = shared-variable "我的电脑\\Global.lvlib\\传感器码-左"() -> (w300:string)  [unwired: 1 in, 1 out]
                        n265 = call "Report.vi"("文件重命名"=TRUE, "文件名称"=w300, "检测结果"="判定结果") -> ("PRODUCT_VAULE"=w302:string)  [unwired: 7 in, 1 out]
                      }
                      frame #1 {
                        n266 = global read "Global1.vi" "联机模式"() -> (w304:enum16{"单机", "追溯"})
                        n267 = case shown="\"追溯\"" w304 {
                          tunnel: w305 -> [_ w309]
                          frame "单机", Default {
                          }
                          frame "追溯" {
                            n268 = global read "Global.vi" "Result"() -> (w313:refnum<vi>)
                            n269 = property class="Tbl"(reference=w313) -> (reference out=w312:refnum<vi>, "Row Headers[]"=w310:string[])  [unwired: 1 in, 1 out]
                            n270 = property class="Tbl"(reference=w312) -> ("Value"=w311:string[][])  [unwired: 1 in, 2 out]
                            n271 = for {
                              tunnel: w311 -> [w317] mode=indexing
                              tunnel: w310 -> [w318] mode=indexing
                              tunnel: [w315] -> w307 mode=indexing if=w316
                              n272 = Build Array (concatenate)(w318, w317) -> (w315:string[])
                              n273 = Index Array(array=w317) -> (element=w319:string)  [unwired: 1 in]
                              n274 = case shown="\"\"" w319 {
                                tunnel: [TRUE FALSE] -> w316
                                frame Default {
                                }
                                frame "" {
                                }
                              }
                            }
                            n275 = global read "追溯Global.vi" "DEVICE_ID"() -> (w308:string)
                            n276 = global read "追溯Global.vi" "USER_ID"() -> (w314:string)
                            n277 = local read "左code"() -> (w306:string)
                            n278 = call "UPRESULT.vi"("DEVICE_ID"=w308, "USER_ID"=w314, "CODE_ID"=w306, "RESULT_VALUE"=w309) -> ()  [unwired: 11 in, 1 out]
                            n279 = call "UPTEST.vi"("Result"=w307, "CODE_ID"=w306, "DEVICE_ID"=w308) -> ()  [unwired: 6 in, 1 out]
                          }
                        }
                      }
                      frame #2 {
                        n280 = Wait (ms)(milliseconds to wait=u32 50 ("等待时间（毫秒）")) -> ()  [unwired: 1 out]
                      }
                    }
                  }
                  frame #1 {
                    n281 = disable-structure shown="禁用" {
                      frame Disabled {
                        n282 = call "左工位状态.vi"("枚举"=enum16{"Read", "Write"}."Write", "Status_Write"=i16 3) -> ()  [unwired: 9 in, 1 out]
                      }
                      frame Enabled {
                      }
                    }
                    n283 = global write "Global.vi" "计时开始"(FALSE ("计时开始")) -> ()
                  }
                  frame #2 {
                    n284 = local write "STEP"("进入自动" ("STEP")) -> ()
                  }
                }
              }
            }
          }
        }
        n285 = Wait (ms)(milliseconds to wait=u32 10 ("等待时间（毫秒）")) -> ()  [unwired: 1 out]
        n286 = global read "Global.vi" "程序关闭"() -> (w14:bool)
      }
    }
  }
